vi "Init.vi"(8 "error in (no error)":errorcluster caption="entrée d'erreur (pas d'erreur)", 11 "Cryptographic Hash_SHA256 en entrée":refnum<class "Cryptographic Hash_SHA256.lvclass">) -> (0 "error out":errorcluster caption="sortie d'erreur", 3 "Cryptographic Hash_SHA256 en sortie":refnum<class "Cryptographic Hash_SHA256.lvclass">)   [LabVIEW 2020, in "Library Cryptographic Hash.lvlib" / "Cryptographic Hash_SHA256.lvclass"]
uses:
  Cryptographic Hash_SHA256.lvclass
  Cryptographic Hash_SHA256.lvclass/Cryptographic Hash_SHA256.ctl
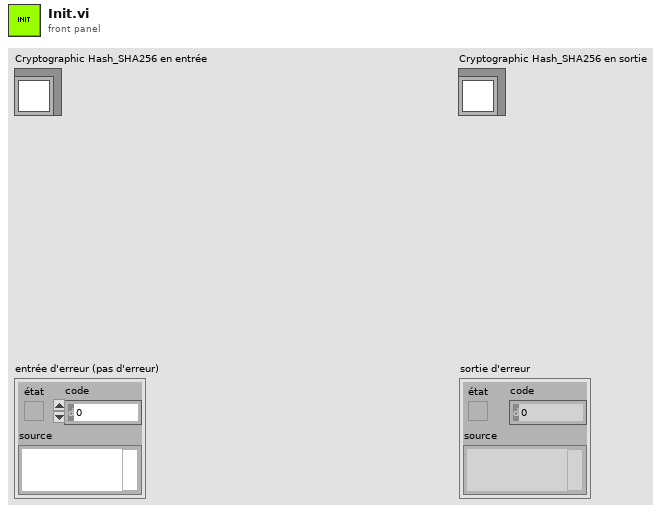
[diagram p1: front panel]
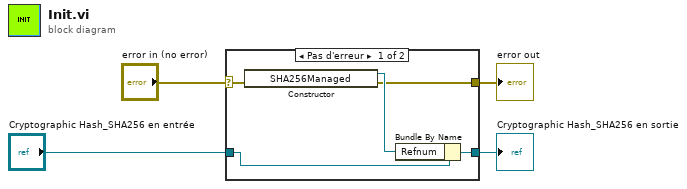
[diagram p0: block diagram]
diagram:
  n1 = case shown="Pas d'erreur" "error in (no error)" {
    selector: "error in (no error)" -> [w6 w11]
    tunnel: [w5 w11] -> w3
    tunnel: [w9 w10] -> w1
    tunnel: "Cryptographic Hash_SHA256 en entrée" -> [w7 w10]
    frame No Error {
      n2 = constructor class="SHA256Managed"(error in=w6) -> (reference out=w8:refnum<k24>, error out=w5:errorcluster)  [unwired: 2 in, 1 out]
      n3 = Bundle By Name(cluster=w7, "Refnum"=w8) -> (w9:refnum<class "Cryptographic Hash_SHA256.lvclass">)
    }
    frame Error {
    }
  }
  "error out" <- w3
  "Cryptographic Hash_SHA256 en sortie" <- w1
